vi "Intensity Graph.vi"() -> ()   [LabVIEW 2011]
panel:
  in  "multiplier":dbl
  out "j":i32
  in  "Grid Spacing":dbl
  out "i":i32
  in  "N":i32
  out "Intensity Graph":dbl[][](graph)
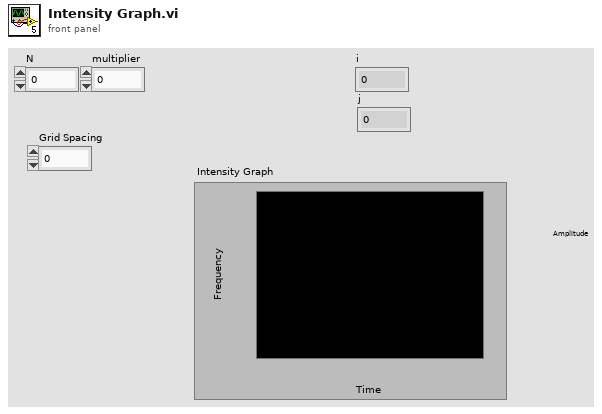
[diagram p1: front panel]
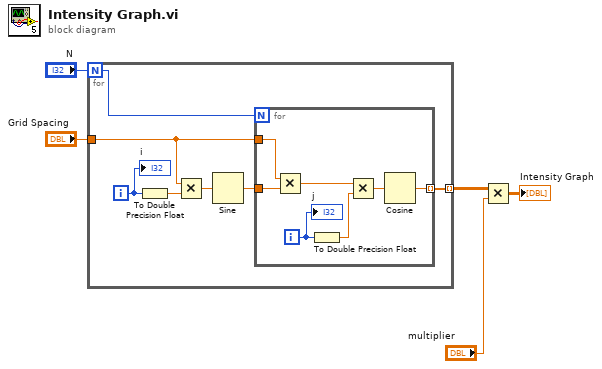
[diagram p0: block diagram]
diagram:
  n1 = for {
    N: "N" -> [w8]
    tunnel: "Grid Spacing" -> [w9]
    tunnel: [w6] -> w2 mode=indexing
    i -> [w12]
    n2 = To Double Precision Float(number=w12) -> (double precision float=w11:dbl)
    n3 = Multiply(x=w9, y=w11) -> (x*y=w10:dbl)
    n4 = Sine(x=w10) -> (sin(x)=w7:dbl)
    n5 = for {
      N: w8 -> [_]
      tunnel: w9 -> [w18]
      tunnel: w7 -> [w17]
      tunnel: [w13] -> w6 mode=indexing
      i -> [w19]
      n6 = Multiply(x=w18, y=w17) -> (x*y=w15:dbl)
      n7 = To Double Precision Float(number=w19) -> (double precision float=w16:dbl)
      n8 = Multiply(x=w15, y=w16) -> (x*y=w14:dbl)
      n9 = Cosine(x=w14) -> (cos(x)=w13:dbl)
      "j" <- w19
    }
    "i" <- w12
  }
  n10 = Multiply(x=w2, y="multiplier") -> (x*y=→"Intensity Graph":dbl[][])
